vi "downconvert_test.vi"() -> ()   [LabVIEW 2025]
uses:
  <instrlib>/_niInstr/DSP/v1/Shared/Public/IQ Data.ctl
  <instrlib>/_niInstr/DSP/v1/Shared/niInstr DSP v1 Shared.lvlib
panel:
  out "Waveform Graph":i16[](graph)
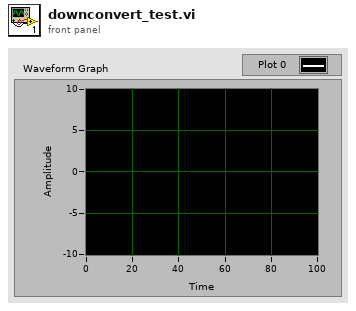
[diagram p1: front panel]
types:
  T1 = typedef "niInstr DSP v1 Shared.lvlib/IQ Data.ctl" = cluster{"I":fxp<+/-,18,1>, "Q":fxp<+/-,18,1>, "overflow":bool}
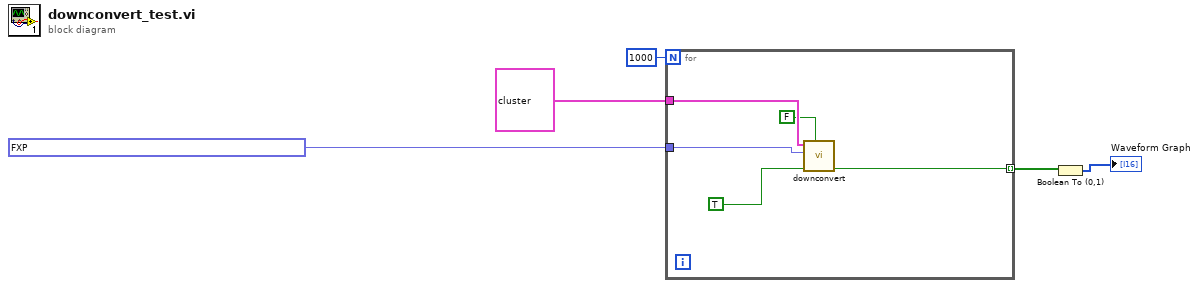
[diagram p0: block diagram]
diagram:
  n1 = for {
    N: 1000 -> [_]
    tunnel: fxp<+,48,1> 0.008000000000002672 ("output sample rate") -> [w9]
    tunnel: T1[] [{"I"=0.0, "Q"=0.0, "overflow"=FALSE}, {"I"=0.0, "Q"=0.0, "overflow"=FALSE}, {"I"=0.0, "Q"=0.0, "overflow"=FALSE}, {"I"=0.0, "Q"=0.0, "overflow"=FALSE}] ("data in") -> [w8]
    tunnel: [w6] -> w3 mode=indexing
    n2 = call "downconvert.vi"("reset"=FALSE, "input valid"=TRUE, "output sample rate"=w9, "data in"=w8) -> ("output valid"=w6:bool)  [unwired: 6 in, 1 out]
  }
  n3 = Boolean To (0,1)(Boolean=w3) -> (0, 1=→"Waveform Graph":i16[])
